vi "LinearFilter_Calculate.vi"(9 "Input":dbl format="%13.5p", 11 "In LINEAR_FILTER":T1 {"Outputs" format="%13.5g"; "Inputs" format="%13.5g"; "OutputGains" format="%13.5g"; "InputGains" format="%13.5g"}) -> (1 "Output":dbl format="%13.5p", 3 "Out LINEAR_FILTER":T1 {"Outputs" format="%13.5g"; "Inputs" format="%13.5g"; "OutputGains" format="%13.5g"; "InputGains" format="%13.5g"})   [LabVIEW 2023]
doc: "Calculates the next value of the filter. To work correctly this must be called periodically\n\nInputs:\n - inLinearfilter - Linear filter data structure\n - input - Current input value.\n \nOutputs:\n - outLinearfilter - Updated linear filter data structurea\n - output - The filtered value at this step"
uses:
  <vilib>/Rock Robotics/WPI/ThirdParty/JAS_Junk/TrajLib/TypeDef/LINEAR_FILTER.ctl
  <vilib>/Rock Robotics/WPI/ThirdParty/JAS_Junk/TrajLib/Trajectory_Library.lvlib
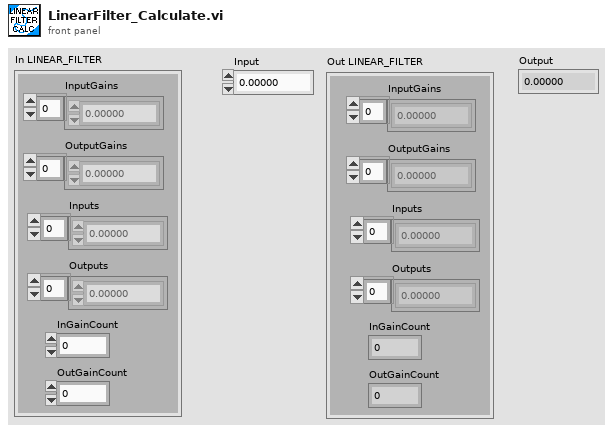
[diagram p1: front panel]
types:
  T1 = typedef "Trajectory_Library.lvlib/LINEAR_FILTER.ctl" = cluster{"InputGains":dbl[], "OutputGains":dbl[], "Inputs":dbl[], "Outputs":dbl[], "InGainCount":i32, "OutGainCount":i32}
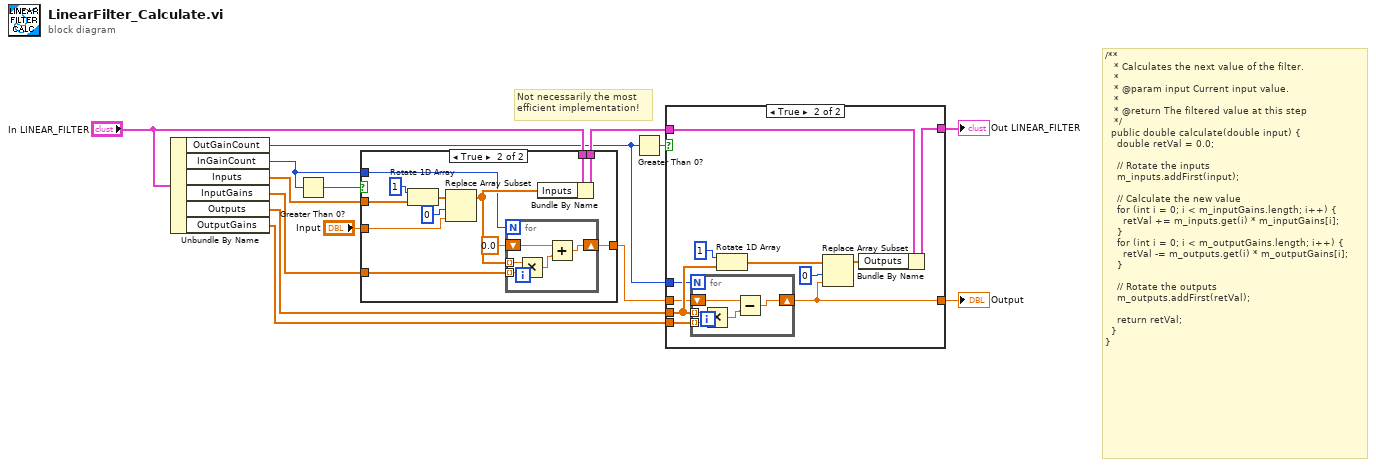
[diagram p0: block diagram]
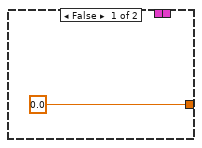
[diagram p3: hidden frame]
diagram:
  # "Not necessarily the most\nefficient implementation!"
  # "/**\n   * Calculates the next value of the filter.\n   *\n   * @param input Current input value.\n   *\n   * @return The filtered value at this step\n   */\n  public double calculate(double input) {\n    double retVal = 0.0;\n\n    // Rotate the inputs\n    m_inputs.addFirst(input);\n\n    // Calculate the new value\n    for (int i = 0; i < m_inputGains.length; i++) {\n      retVal += m_inputs.get(i) * m_inputGains[i];\n    }\n    for (int i = 0; i < m_outputGains.length; i++) {\n      retVal -= m_outputs.get(i) * m_outputGains[i];\n    }\n\n    // Rotate the outputs\n    m_outputs.addFirst(retVal);\n\n    return retVal;\n  }\n}"
  n1 = Unbundle By Name("In LINEAR_FILTER") -> ("OutGainCount"=w1:i32, "InGainCount"=w2:i32, "Inputs"=w12:dbl[], "InputGains"=w9:dbl[], "Outputs"=w11:dbl[], "OutputGains"=w8:dbl[])
  n2 = Greater Than 0?(x=w2) -> (x > 0?=w14:bool)
  n3 = case shown="True" w14 {
    tunnel: w12 -> [_ w26]
    tunnel: "Input" -> [_ w23]
    tunnel: w9 -> [_ w18]
    tunnel: "In LINEAR_FILTER" -> [w16 w28]
    tunnel: [w16 w27] -> w6
    tunnel: [0.0 w20] -> w4
    tunnel: w2 -> [_ w17]
    frame False {
    }
    frame True {
      n4 = Rotate 1D Array(1:w26, 2:1 ("n")) -> (0:w24:dbl[])
      n5 = Replace Array Subset(array=w24, new element=w23, index=0) -> (w19:dbl[])
      n6 = for {
        N: w17 -> [_]
        shift-right: [w33] -> w20
        shift-left: 0.0 -> [w32]
        tunnel: w19 -> [w30] mode=indexing
        tunnel: w18 -> [w29] mode=indexing
        n7 = Multiply(x=w30, y=w29) -> (x*y=w31:dbl)
        n8 = Add(x=w32, y=w31) -> (x+y=w33:dbl)
      }
      n9 = Bundle By Name(cluster=w28, "Inputs"=w19) -> (w27:T1)
    }
  }
  n10 = Greater Than 0?(x=w1) -> (x > 0?=w13:bool)
  n11 = case shown="True" w13 {
    tunnel: w11 -> [_ w39]
    tunnel: w8 -> [_ w38]
    tunnel: w6 -> [w35 w46]
    tunnel: [w35 w45] -> w5
    tunnel: w4 -> [w34 w37]
    tunnel: [w34 w40] -> w3
    tunnel: w1 -> [_ w36]
    frame False {
    }
    frame True {
      n12 = for {
        N: w36 -> [_]
        shift-right: [w51] -> w40
        shift-left: w37 -> [w50]
        tunnel: w39 -> [w48] mode=indexing
        tunnel: w38 -> [w47] mode=indexing
        n13 = Multiply(x=w48, y=w47) -> (x*y=w49:dbl)
        n14 = Subtract(x=w50, y=w49) -> (x-y=w51:dbl)
      }
      n15 = Rotate 1D Array(1:w39, 2:1 ("n")) -> (0:w43:dbl[])
      n16 = Replace Array Subset(array=w43, new element=w40, index=0) -> (w41:dbl[])
      n17 = Bundle By Name(cluster=w46, "Outputs"=w41) -> (w45:T1)
    }
  }
  "Out LINEAR_FILTER" <- w5
  "Output" <- w3
